vi "IsEqual.vi"(2 "is equal to":refnum<class>, 3 "reference in":refnum<class "G#Object.lvclass">) -> (0 "is equal":bool, 1 "reference out":refnum<class "G#Object.lvclass">)   [LabVIEW 2020, in "G#Object.lvclass"]
doc: "Checks if the two input object references are one and the same object."
uses:
  G#Object.lvclass
  G#Object.lvclass/G#Object.ctl
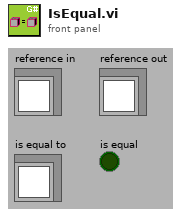
[diagram p1: front panel]
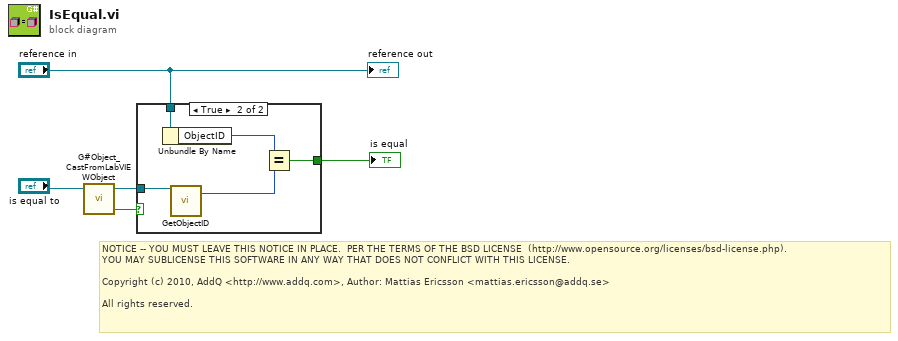
[diagram p0: block diagram]
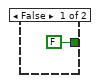
[diagram p2: hidden frame]
diagram:
  # "NOTICE -- YOU MUST LEAVE THIS NOTICE IN PLACE.  PER THE TERMS OF THE BSD LICENSE  (http://www.opensource.org/licenses/bsd-license.php).\nYOU MAY SUBLICENSE THIS SOFTWARE IN ANY WAY THAT DOES NOT CONFLICT WITH THIS LICENSE.\n\nCopyright (c) 2010, AddQ <http://www.addq.com>, Author: Mattias Ericsson <mattias.ericsson@addq.se>\n\nAll rights reserved."
  n1 = call "G#Object_CastFromLabVIEWObject.vi"("LabVIEWObject in"="is equal to") -> ("is of G#Object?"=w1:bool, "reference out"=w2:refnum<class "G#Object.lvclass">)  [unwired: 2 in, 1 out]
  n2 = case shown="True" w1 {
    tunnel: [FALSE w11] -> w5
    tunnel: "reference in" -> [_ w9]
    tunnel: w2 -> [_ w7]
    frame False {
    }
    frame True {
      n3 = Unbundle By Name(w9) -> ("ObjectID"=w10:u32)
      n4 = call-dynamic "GetObjectID.vi"("reference in"=w7) -> ("object ID"=w8:u32)  [unwired: 16 in, 2 out]
      n5 = Equal?(x=w10, y=w8) -> (x = y?=w11:bool)
    }
  }
  "is equal" <- w5
  "reference out" <- "reference in"
